vi "Handle setConfiguration.vi"(8 "error in (no error)":errorcluster, 10 "setConfiguration":variant, 11 "Instrument.Template in":refnum<class "Instrument.Template.lvclass">) -> (0 "error out":errorcluster, 3 "Instrument.Template out":refnum<class "Instrument.Template.lvclass">)   [LabVIEW 2019, in "Instrument.Template.lvclass"]
uses:
  Instrument.Template.lvclass
  Instrument.Template.lvclass/Instrument.Template.ctl
  45e4b271-6884-462c-ad3a-d505ab08eb62.vi
  45e4b271-6884-462c-ad3a-d505ab08eb62.vi/33cca3f2-92f2-4575-9ff1-f52ec6854787.vi
  45e4b271-6884-462c-ad3a-d505ab08eb62.vi/99a44749-528d-4add-be62-6bd77fc5e803.vi
  <vilib>/Utility/Data Type/Get Type Information.vi
  <vilib>/JDP Science/JSONtext/JSON text to Variant.vi
  <vilib>/JDP Science/JSONtext/LVClass Serializer/JSONtext LVClass Serializer.lvclass
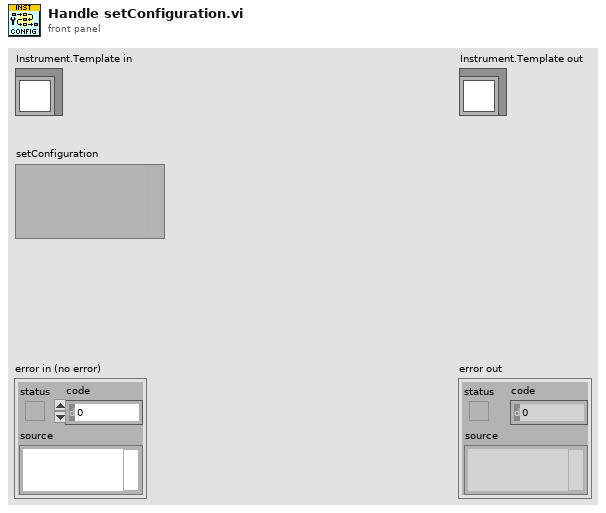
[diagram p1: front panel]
types:
  T1 = typedef "Instrument.Template.lvclass/Instrument.Template.Configuration--Cluster.ctl" = cluster{"Example Setting 1":dbl, "Example Setting 2":dbl, "Example Setting 3":string}
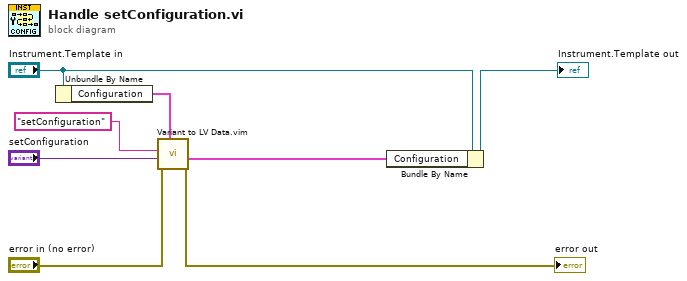
[diagram p0: block diagram]
diagram:
  n1 = Unbundle By Name("Instrument.Template in") -> ("Configuration"=w7:T1)
  n2 = call "Variant to LV Data.vim"("type"=w7, "error in (no error)"="error in (no error)", "JSON Data in"="setConfiguration", "Command"="setConfiguration") -> ("error out"=→"error out":errorcluster, "Data out"=w1:T1)  [unwired: 4 in, 2 out]
  n3 = Bundle By Name(cluster="Instrument.Template in", "Configuration"=w1) -> (→"Instrument.Template out":refnum<class "Instrument.Template.lvclass">)
